vi "Execute Term Handle.vi"(4 "Menu Item Tag Suffix":string, 8 "错误输入（无错误）":errorcluster, 11 "接线端输入":refnum<vi>) -> (0 "错误输出":errorcluster)   [LabVIEW 2020]
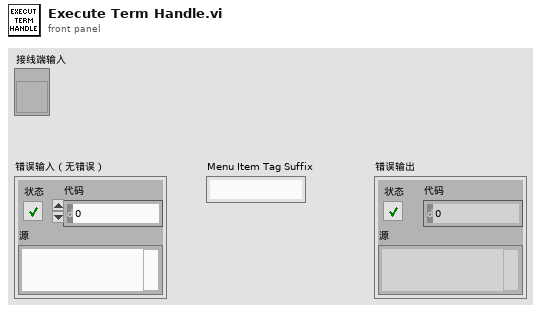
[diagram p1: front panel]
types:
  T1 = typedef "LVRectTypeDef.ctl" = cluster{"Left":i16, "Top":i16, "Right":i16, "Bottom":i16}
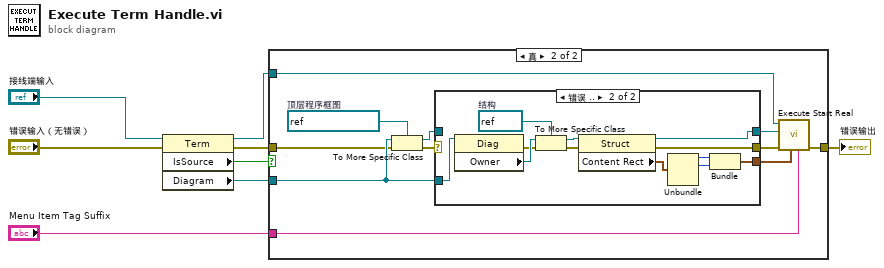
[diagram p0: block diagram]
diagram:
  n1 = property class="Term"(reference="接线端输入", error in="错误输入（无错误）") -> (reference out=w4:refnum<vi>, error out=w8:errorcluster, "IsSource"=w2:bool, "Diagram"=w3:refnum<vi>)
  n2 = case shown="真" w2 {
    tunnel: w3 -> [_ w17]
    tunnel: w4 -> [_ w20]
    tunnel: "Menu Item Tag Suffix" -> [_ w14]
    tunnel: [w9 w11] -> w7
    tunnel: w8 -> [w9 w10]
    frame False {
    }
    frame True {
      w19 = refnum<vi> refnum  # 顶层程序框图
      n3 = To More Specific Class(target class=w19, reference=w17, error in=w10) -> (specific class reference=w15:refnum<vi>, error out=w18:errorcluster)
      n4 = case shown="错误 .." w18 {
        selector: w18 -> [w21 _]
        tunnel: w17 -> [_ w34]
        tunnel: [_ w26] -> w13
        tunnel: [w22 w27] -> w16
        tunnel: w15 -> [w22 _]
        tunnel: [w21 w23] -> w12
        frame No Error {
        }
        frame Error {
          w33 = refnum<vi> refnum  # 结构
          n5 = property class="Diag"(reference=w34) -> (error out=w25:errorcluster, "Owner"=w32:refnum<vi>)  [unwired: 1 in, 1 out]
          n6 = To More Specific Class(target class=w33, reference=w32, error in=w25) -> (specific class reference=w31:refnum<vi>, error out=w24:errorcluster)
          n7 = property class="Struct"(reference=w31, error in=w24) -> (reference out=w27:refnum<vi>, error out=w23:errorcluster, "Content Rect"=w28:T1)
          n8 = Unbundle(w28) -> ("Left"=w30:i16, "Top"=w29:i16)  [unwired: 2 out]
          n9 = Bundle("Left"=w30, "Top"=w29) -> (w26:cluster{"Left":i16, "Top":i16})  [unwired: 1 in]
        }
      }
      n10 = call "Execute Start Real.vi"("Menu Item Tag Suffix"=w14, "相对位置原点"=w13, "错误输入（无错误）"=w12, "所有者引用句柄"=w16, "接线端输入"=w20) -> ("错误输出"=w11:errorcluster)  [unwired: 6 in]
    }
  }
  "错误输出" <- w7
